vi "Help.vi"() -> ()   [LabVIEW 2020]
panel:
  in  "停止":bool
  # "璐宝宝最可爱~"
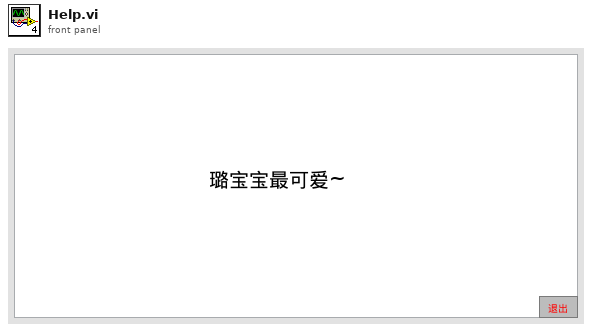
[diagram p1: front panel]
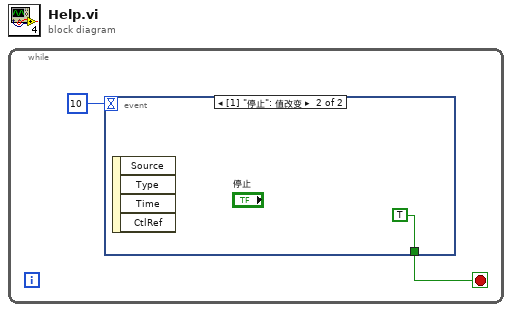
[diagram p0: block diagram]
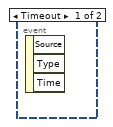
[diagram p2: hidden frame]
diagram:
  n1 = while {
    stop <- w1 stop-if-true
    n2 = event shown="[1] \"停止\": 值改变" {
      selector: _ -> [_ _]
      dyn-events: _ -> [_ _]
      timeout: 10 -> [_ _]
      tunnel: [_ TRUE] -> w1
      event Timeout {
        n3 = event-data() -> ()  [unwired: 1 in, 3 out]
      }
      event "停止": Value Change {
        n4 = event-data() -> ()  [unwired: 1 in, 4 out]
      }
    }
  }
